vi "Log Entry Creator.vi"(8 "error in (no error)":errorcluster, 10 "Signal Integration Values":dbl[](array[numeric]), 11 "Waveforms":waveform(dbl)[](array[waveform])) -> (0 "error out":errorcluster, 3 "Log Entry":string)   [LabVIEW 2013, in "Breakdown Acoustics Controls.lvlib"]
uses:
  Breakdown Acoustics Controls.lvlib
  <vilib>/Waveform/WDTOps.llb/WDT Index Channel DBL.vi
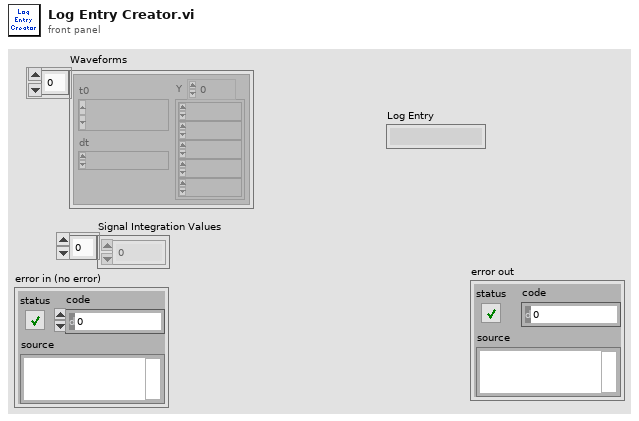
[diagram p1: front panel]
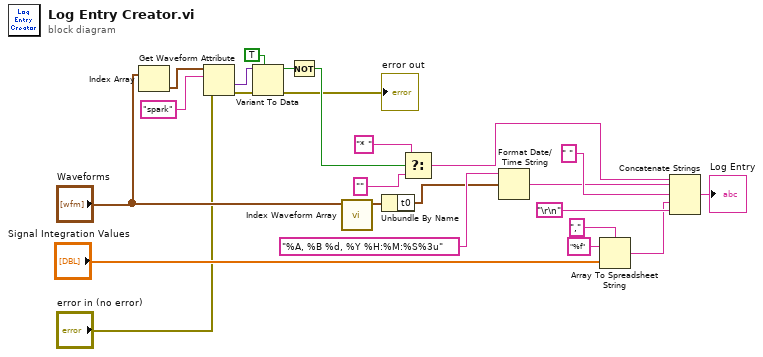
[diagram p0: block diagram]
diagram:
  n1 = Index Array(array="Waveforms") -> (element=w10:waveform(dbl))  [unwired: 1 in]
  n2 = Get Waveform Attribute(4:"error in (no error)", 6:"spark" ("name"), 7:w10) -> (0:w8:errorcluster, 1:w9:variant)  [unwired: 1 in, 2 out]
  n3 = Variant To Data(error in=w8, type=TRUE, Variant=w9) -> (data=w4:bool, error out=→"error out":errorcluster)
  n4 = Not(x=w4) -> (.not. x?=w3:bool)
  n5 = call-poly <vilib>:"Index Waveform Array.vi"("waveform array"="Waveforms") -> ("waveform"=w17:waveform(dbl))  [unwired: 9 in, 1 out]
  n6 = Unbundle By Name(w17) -> ("t0"=w14:timestamp)
  n7 = Select(t="* ", s=w3, f="") -> (s? t:f=w13:string)
  n8 = Format Date/Time String(time format string (%c)="%A, %B %d, %Y %H:%M:%S%3u", seconds (now)=w14) -> (date/time string=w15:string)  [unwired: 1 in]
  n9 = Array To Spreadsheet String(delimiter (Tab)=",", array="Signal Integration Values", 3:"%f" ("format string")) -> (spreadsheet string=w22:string)
  n10 = Concatenate Strings(w13, w15, " ", w22, "\r\n") -> (→"Log Entry":string)
